vi "RunIndicator.vi"(2 "Step":enum16{"Open", "Close"}(ring), 5 "reference":refnum<k24>, 11 "error in (no error)":errorcluster) -> (15 "error out":errorcluster)   [LabVIEW 2011]
uses:
  System.Windows.Forms
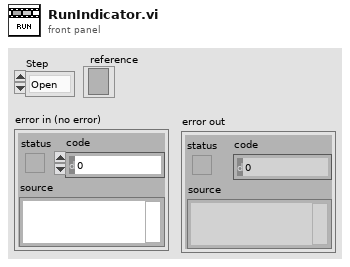
[diagram p1: front panel]
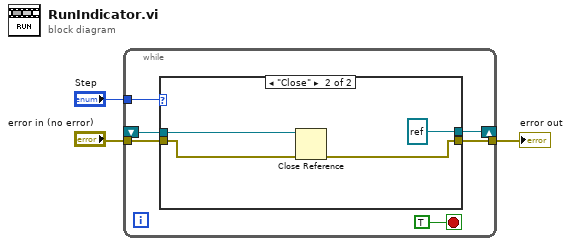
[diagram p0: block diagram]
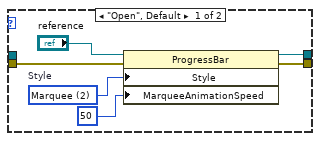
[diagram p2: hidden frame]
diagram:
  n1 = while {
    shift-right: [w9] -> _
    shift-left: _ -> [w7]
    tunnel: "Step" -> [w8]
    tunnel: "error in (no error)" -> [w6]
    tunnel: [w5] -> w1
    stop <- TRUE stop-if-true
    n2 = case shown="\"Close\"" w8 {
      tunnel: [w12 refnum<k24> refnum ("reference")] -> w9
      tunnel: w7 -> [_ w19]
      tunnel: w6 -> [w11 w17]
      tunnel: [w10 w18] -> w5
      frame "Open", Default {
        w14 = 2 items=["Blocks", "Continuous", "Marquee"]  # Style
        n3 = property class="ProgressBar"(reference="reference", error in=w11, "Style"=w14, "MarqueeAnimationSpeed"=50) -> (reference out=w12:refnum<k24>, error out=w10:errorcluster)
      }
      frame "Close" {
        n4 = Close Reference(reference=w19, error in (no error)=w17) -> (error out=w18:errorcluster)
      }
    }
  }
  "error out" <- w1
